vi "DM Message Loop.vi"(8 "error in (no error)":errorcluster, 9 "Data Queue":refnum<queue>, 10 "Data Notifier":refnum<notifier>, 11 "Message Queues":T1) -> (0 "error out":errorcluster)   [LabVIEW 2015, in "DM.lvlib"]
uses:
  DM.lvlib
  support/Message Queue/All Message Queues.ctl
  support/Message Queue/Message Cluster.ctl
  DM Configuration.ctl
  DM State.ctl
  DM Loop State.ctl
  <vilib>/Utility/error.llb/Error Cluster From Error Code.vi
  <vilib>/Utility/file.llb/Read Delimited Spreadsheet (DBL).vi
  <vilib>/ErrorRing/Error Ring.xnode
  support/Message Queue/Message Queue.lvlib
  <userlib>/BMC/BMC.lvlib
panel:
  out "file (use dialog)":path=path "X:/Lab/Equipment/Boston Micromachines Multi-DM/Flash-Drive Contents/C187W147#040_Flat_Map/18W147#040_CLOSED_LOOP_VOLTAGES.txt"
  out "Intensity Graph":dbl[][](graph)
  in  "blank":dbl[](array[slide]) scale=-1.0..1.0
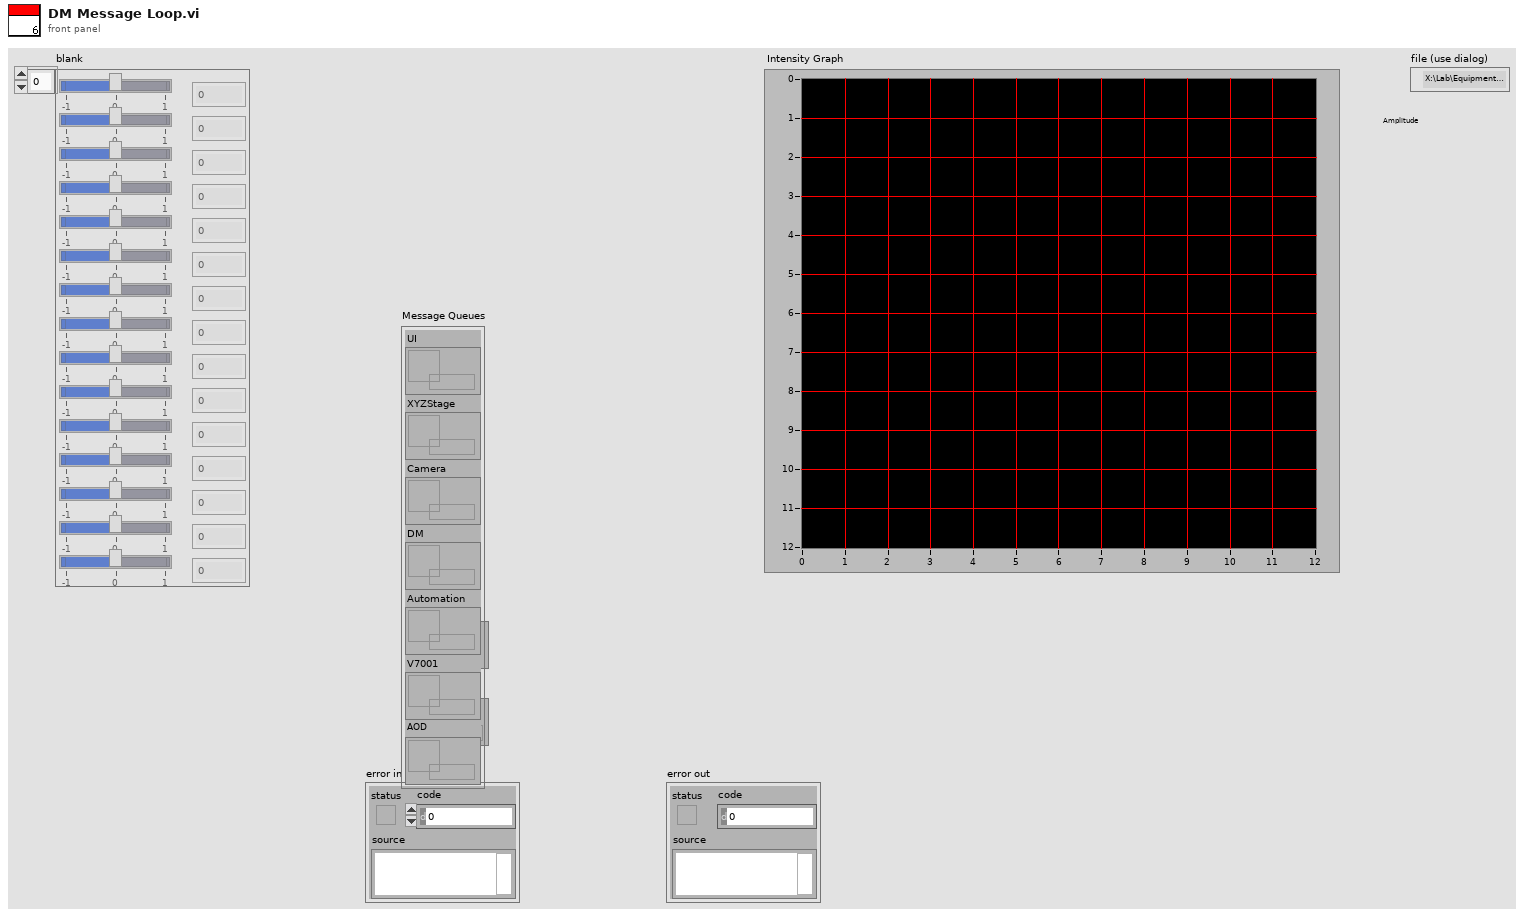
[diagram p1: front panel]
types:
  T1 = typedef "Message Queue.lvlib/All Message Queues.ctl" = cluster{"UI":refnum<queue>, "XYZStage":refnum<queue>, "Camera":refnum<queue>, "DM":refnum<queue>, "Automation":refnum<queue>, "V7001":refnum<queue>, "AOD":refnum<queue>}
  T2 = typedef "DM.lvlib/DM State.ctl" = cluster{"DM State":T3, "Last Image Sent":dbl[][], "Flatmap":dbl[], "Flatmap Path":path, "Matlab Directory Path":path}
  T3 = typedef "DM.lvlib/DM Loop State.ctl" = enum16{"Idle", "Connected"}
  T4 = typedef "DM.lvlib/DM Configuration.ctl" = cluster{"Selected Profile":string, "dm out":cluster{"type":i32, "ID":i32, "size":i32, "@dummy control@":i8, "@dummy control@":i8, "@dummy control@":i8, "@dummy control@":i8, "lutName":u64}}
  T5 = cluster{"type":i32, "ID":i32, "size":i32, "@dummy control@":i8, "@dummy control@":i8, "@dummy control@":i8, "@dummy control@":i8, "lutName":u64}
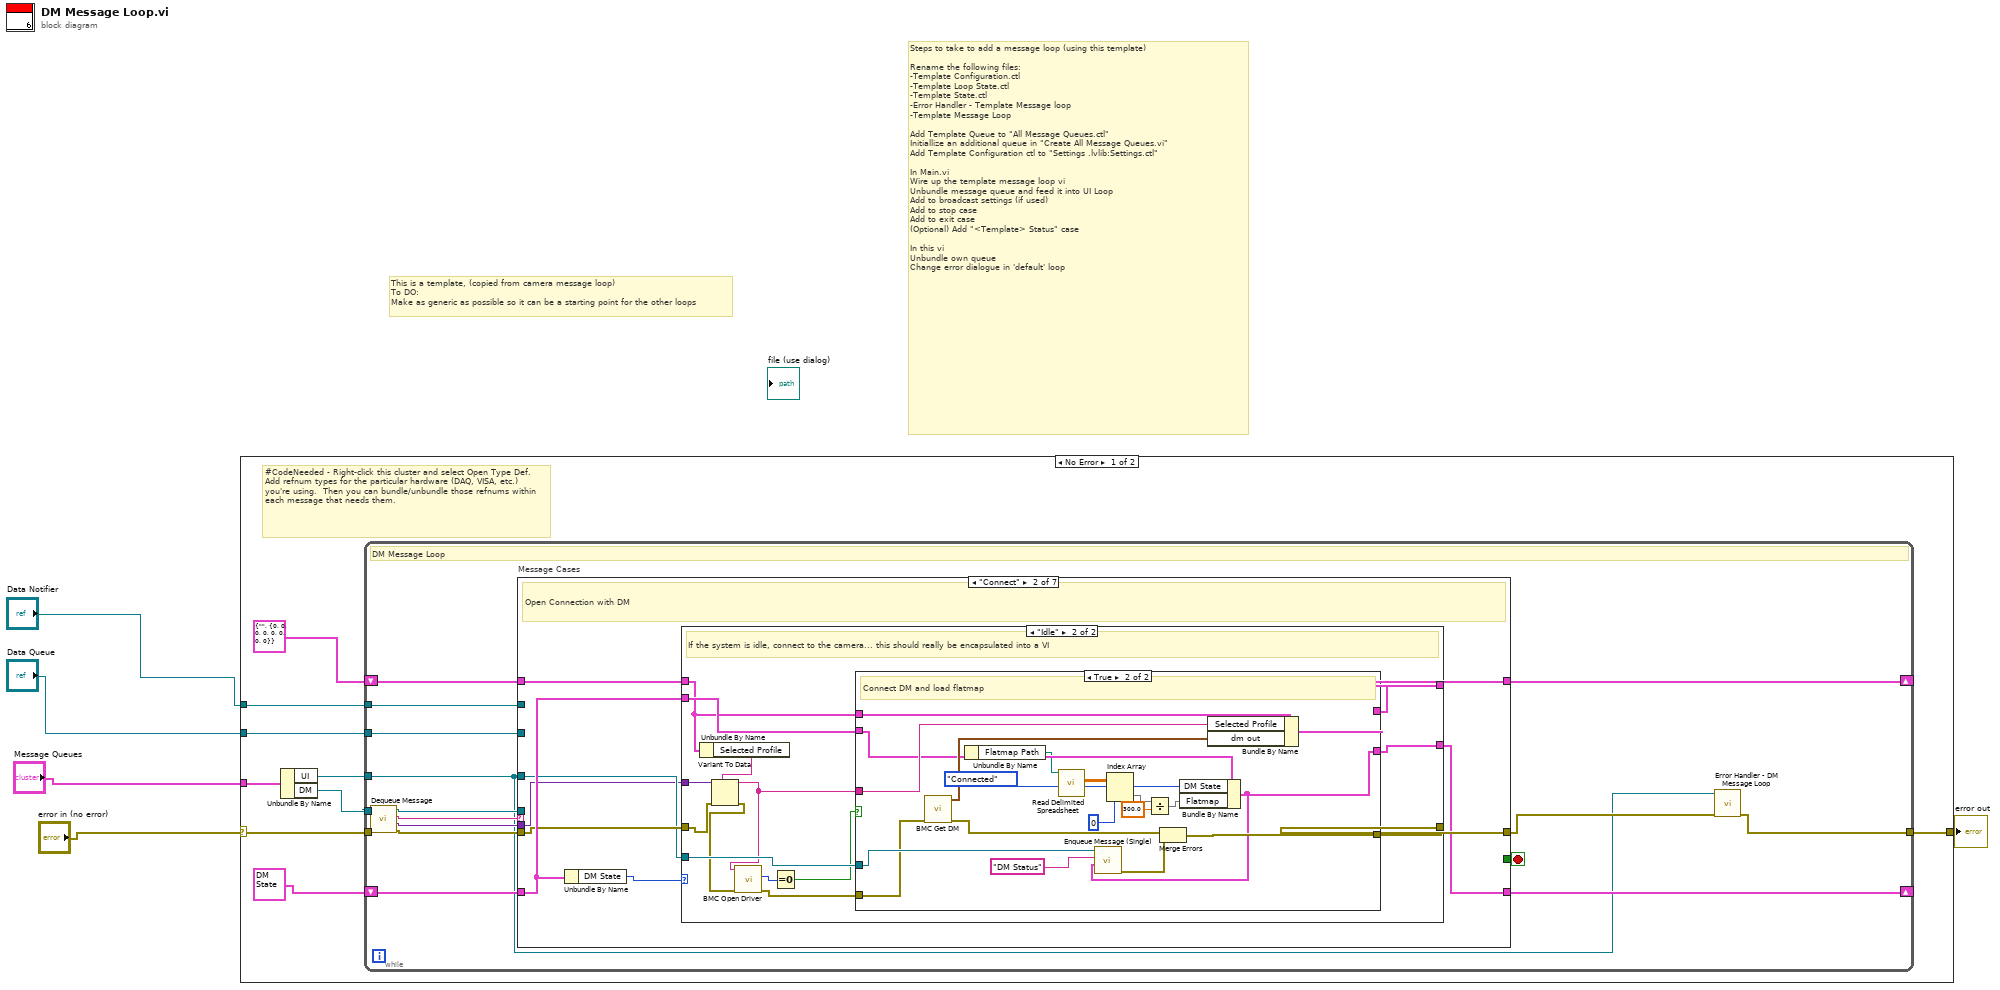
[diagram p0: block diagram]
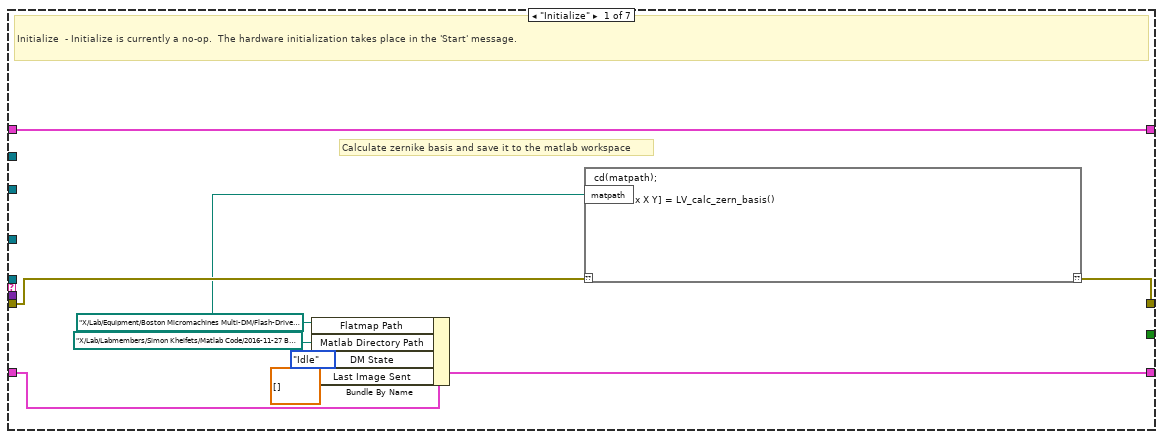
[diagram p2: hidden frame]
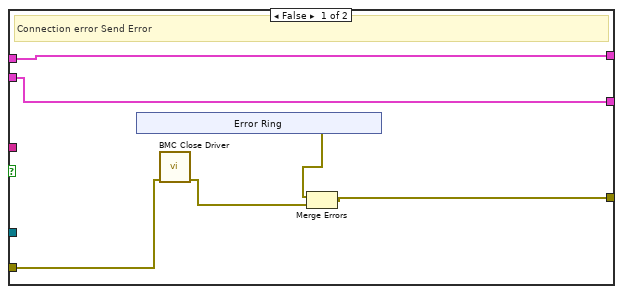
[diagram p4: hidden frame]
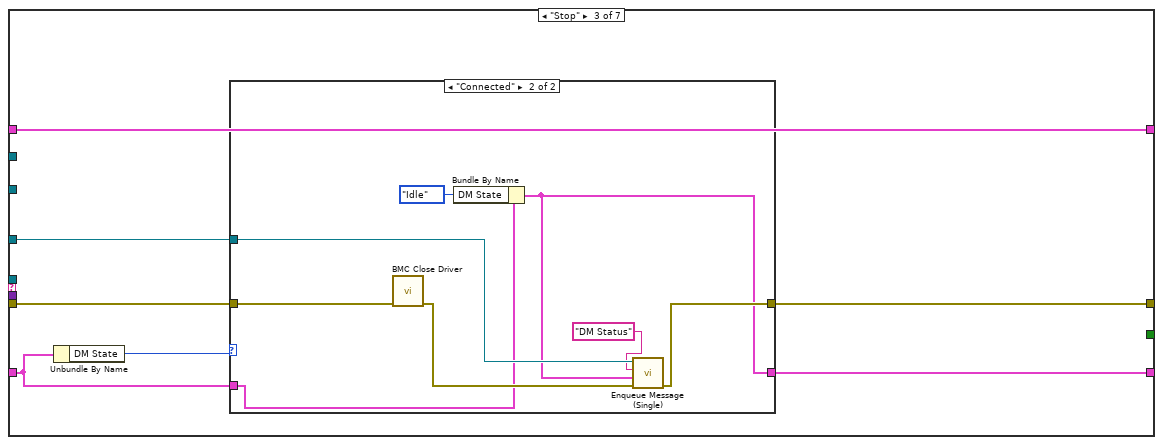
[diagram p5: hidden frame]
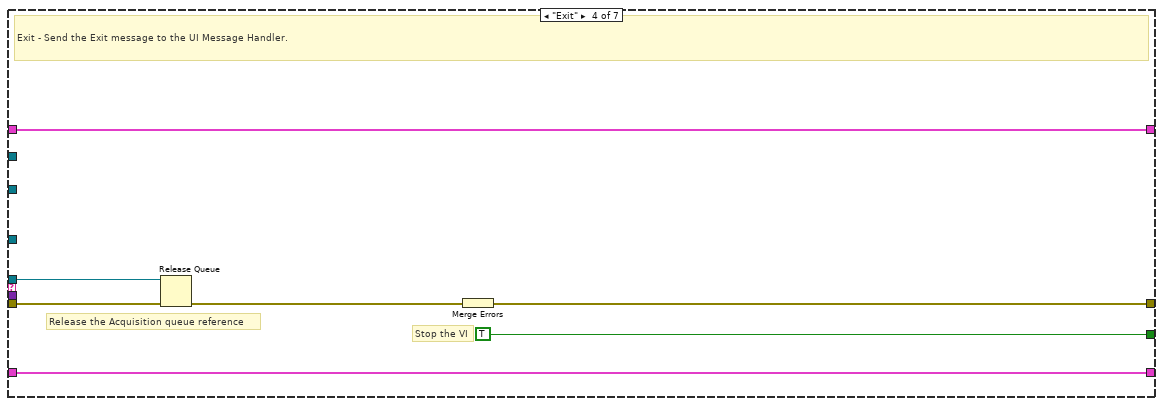
[diagram p7: hidden frame]
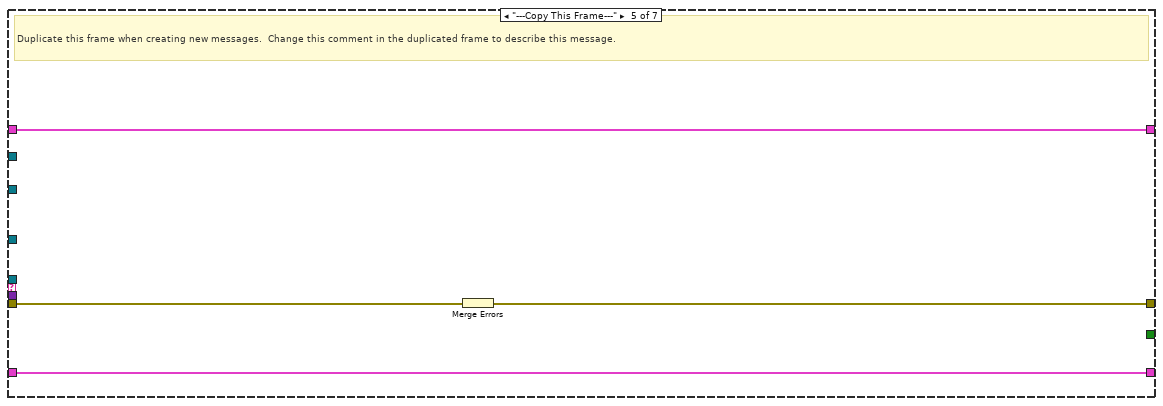
[diagram p8: hidden frame]
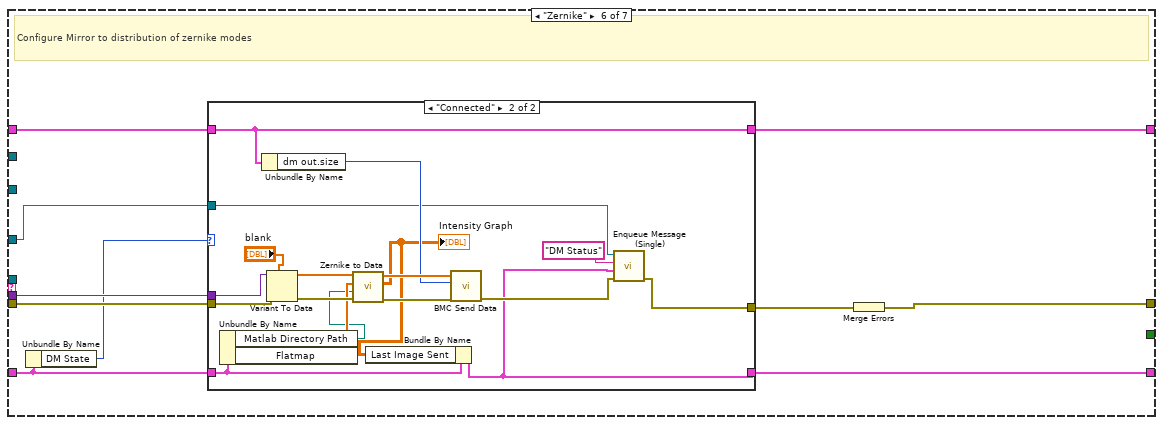
[diagram p9: hidden frame]
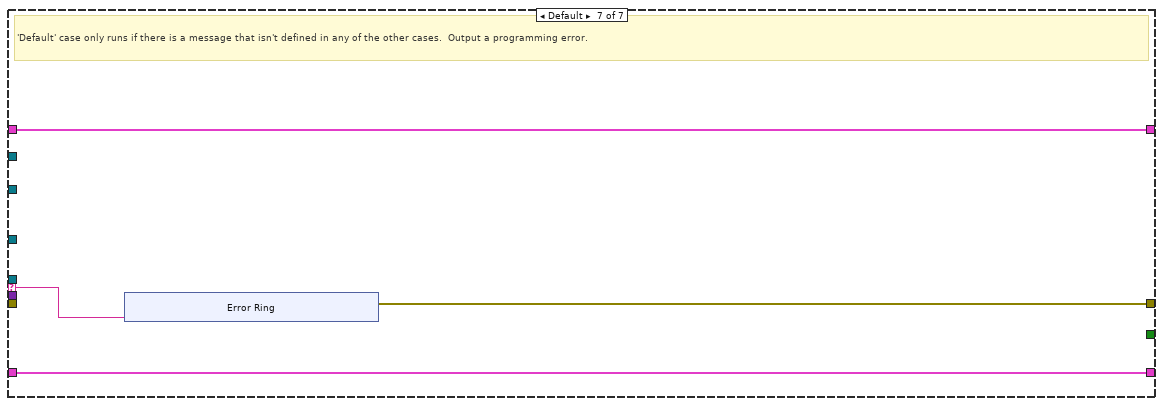
[diagram p11: hidden frame]
diagram:
  # "Steps to take to add a message loop (using this template)\n\nRename the following files:\n-Template Configuration.ctl\n-Template Loop State.ctl\n-Template State.ctl\n-Error Handler - Template Message loop\n-Template Message Loop\n\nAdd Template Queue to \"All Message Queues.ctl\"\nInitiallize an additional queue in \"Create All Message Queues.vi\"\nAdd Template Configuration ctl to \"Settings .lvlib:Settings.ctl\"\n\nIn Main.vi\nWire up the template message loop vi\nUnbundle message queue and feed it into UI Loop\nAdd to broadcast settings (if used)\nAdd to stop case\nAdd to exit case\n(Optional) Add \"<Template> Status\" case\n\nIn this vi\nUnbundle own queue\nChange error dialogue in 'default' loop"
  # "This is a template, (copied from camera message loop)\nTo DO:\nMake as generic as possible so it can be a starting point for the other loops"
  n1 = case shown="No Error" "error in (no error)" {
    selector: "error in (no error)" -> [w11 w166]
    tunnel: "Message Queues" -> [w14 _]
    tunnel: [w12 w166] -> w5
    tunnel: "Data Notifier" -> [w9 _]
    tunnel: "Data Queue" -> [w8 _]
    frame No Error {
      # "#CodeNeeded - Right-click this cluster and select Open Type Def.  Add refnum types for the particular hardware (DAQ, VISA, etc.) you're using.  Then you can bundle/unbundle those refnums within each message that needs them."
      n2 = Unbundle By Name(w14) -> ("UI"=w10:refnum<queue>, "DM"=w13:refnum<queue>)
      n3 = while {
        tunnel: w13 -> [w23]
        shift-right: [w29] -> _
        shift-left: T4 {"Selected Profile"="", "dm out"={"type"=0, "ID"=0, "size"=0, "@dummy control@"=0, "@dummy control@"=0, "@dummy control@"=0, "@dummy control@"=0, "lutName"=0}} ("Hardware Configuration") -> [w30]
        tunnel: w10 -> [w15]
        tunnel: w9 -> [w27]
        tunnel: w8 -> [w26]
        shift-right: [w24] -> _
        shift-left: T2 {"DM State"=enum."Idle", "Last Image Sent"=[], "Flatmap"=[], "Flatmap Path"=path "X:/Lab/Equipment/Boston Micromachines Multi-DM/Flash-Drive Contents/C187W147#040_Flat_Map/18W147#040_CLOSED_LOOP_VOLTAGES.txt", "Matlab Directory Path"=path "X:/Lab/Equipment/Boston Micromachines Multi-DM/Flash-Drive Contents/C187W147#040_Flat_Map/18W147#040_CLOSED_LOOP_VOLTAGES.txt"} ("Cluster") -> [w25]
        tunnel: w11 -> [w22]
        tunnel: [w17] -> w12
        stop <- w28 stop-if-true
        # "DM Message Loop"
        n4 = call "Dequeue Message.vi"("error in (no error)"=w22, "Message Queue"=w23) -> ("error out"=w18:errorcluster, "Message Data"=w19:variant, "Message"=w20:string, "dup Message Queue"=w21:refnum<queue>)  [unwired: 6 in]
        n5 = case "Message Cases" shown="\"Connect\"" w20 {
          selector: w20 -> [_ _ _ _ _ _ w155]
          tunnel: w21 -> [_ _ _ w114 _ _ _]
          tunnel: w18 -> [w34 w45 w100 w116 w123 w131 _]
          tunnel: [w35 w46 w99 w118 w121 w133 w156] -> w16
          tunnel: w30 -> [w39 w44 w102 w117 w122 w130 w158]
          tunnel: [w39 w42 w102 w117 w122 w126 w158] -> w29
          tunnel: [_ _ _ TRUE _ _ _] -> w28
          tunnel: w19 -> [_ w40 _ _ _ w132 _]
          tunnel: w15 -> [_ w41 w98 _ _ w124 _]
          tunnel: w27 -> [_ _ _ _ _ _ _]
          tunnel: w26 -> [_ _ _ _ _ _ _]
          tunnel: w25 -> [w33 w47 w96 w113 w120 w128 w157]
          tunnel: [w38 w43 w97 w113 w120 w129 w157] -> w24
          frame "Initialize" {
            w31 = path "X:/Lab/Labmembers/Simon Kheifets/Matlab Code/2016-11-27 BMC Multi-DM" ("Matlab Directory Path")
            # "Calculate zernike basis and save it to the matlab workspace"
            # "Initialize  - Initialize is currently a no-op.  The hardware initialization takes place in the 'Start' message."
            n6 = Bundle By Name(cluster=w33, "Flatmap Path"=path "X:/Lab/Equipment/Boston Micromachines Multi-DM/Flash-Drive Contents/C187W147#040_Flat_Map/18W147#040_CLOSED_LOOP_VOLTAGES.txt", "Matlab Directory Path"=w31, "DM State"=DM_Loop_State."Idle", "Last Image Sent"=dbl[][] []) -> (w38:T2)
            n7 = script code="cd(matpath);\n\n[basis idx X Y] = LV_calc_zern_basis()"("??"=w34, "matpath"=w31) -> ("??"=w35:errorcluster)
          }
          frame "Connect" {
            # "Open Connection with DM"
            n8 = Unbundle By Name(w47) -> ("DM State"=w48:T3)
            n9 = case shown="\"Idle\"" w48 {
              tunnel: [w51 w65] -> w46
              tunnel: w44 -> [w49 w57]
              tunnel: w45 -> [w51 w54]
              tunnel: [w49 w64] -> w42
              tunnel: [w50 w63] -> w43
              tunnel: w41 -> [_ w62]
              tunnel: w47 -> [w50 w61]
              tunnel: w40 -> [_ w55]
              frame "Connected" {
                # "The system is already acquiring. Ignore the \"Connect\" message."
              }
              frame "Idle" {
                # "If the system is idle, connect to the camera... this should really be encapsulated into a VI"
                n10 = Unbundle By Name(w57) -> ("Selected Profile"=w56:string)
                n11 = Variant To Data(error in=w54, type=w56, Variant=w55) -> (data=w52:string, error out=w53:errorcluster)
                n12 = call <userlib>:"BMC Open Driver.vi"("error in (no error)"=w53, "serial_number"=w52) -> ("error out"=w58:errorcluster, "function return"=w60:i32)  [unwired: 7 in, 1 out]
                n13 = Equal To 0?(x=w60) -> (x = 0?=w59:bool)
                n14 = case shown="True" w59 {
                  tunnel: [w69 w95] -> w65
                  tunnel: w58 -> [w66 w88]
                  tunnel: w57 -> [w71 w87]
                  tunnel: [w71 w86] -> w64
                  tunnel: [w68 w91] -> w63
                  tunnel: w62 -> [_ w94]
                  tunnel: w61 -> [w68 w81]
                  tunnel: w52 -> [_ w84]
                  frame False {
                    # "Connection error Send Error"
                    n15 = xnode "Error Ring"() -> ("error out"=w70:errorcluster)
                    n16 = call <userlib>:"BMC Close Driver.vi"("error in (no error)"=w66) -> ("error out"=w67:errorcluster)  [unwired: 9 in, 1 out]
                    n17 = Merge Errors(w70, w67) -> (w69:errorcluster)
                  }
                  frame True {
                    # "Connect DM and load flatmap"
                    n18 = call <userlib>:"BMC Get DM.vi"("error in (no error)"=w88) -> ("error out"=w89:errorcluster, "dm out"=w85:T5)  [unwired: 7 in, 2 out]
                    n19 = Unbundle By Name(w81) -> ("Flatmap Path"=w80:path)
                    n20 = call-poly <vilib>:"Read Delimited Spreadsheet.vi"("file path (dialog if empty)"=w80) -> ("all rows"=w83:dbl[][])  [unwired: 9 in, 5 out]
                    n21 = Index Array(array=w83, index (col)=0 ("disabled index (col)")) -> (element=w78:dbl[])  [unwired: 1 in]
                    n22 = Divide(x=w78, y=300.0) -> (x/y=w77:dbl[])
                    n23 = Bundle By Name(cluster=w81, "DM State"=DM_Loop_State."Connected", "Flatmap"=w77) -> (w91:T2)
                    n24 = call "Enqueue Message (Single).vi"("Message Data"=w91, "Message"="DM Status", "Message Queue"=w94) -> ("error out"=w92:errorcluster)  [unwired: 7 in, 1 out]
                    n25 = Merge Errors(w89, w92) -> (w95:errorcluster)
                    n26 = Bundle By Name(cluster=w87, "Selected Profile"=w84, "dm out"=w85) -> (w86:T4)
                  }
                }
              }
            }
          }
          frame "Stop" {
            n27 = Unbundle By Name(w96) -> ("DM State"=w101:T3)
            n28 = case shown="\"Connected\"" w101 {
              tunnel: w100 -> [w104 w112]
              tunnel: [w104 w110] -> w99
              tunnel: w98 -> [_ w109]
              tunnel: [w103 w105] -> w97
              tunnel: w96 -> [w103 w107]
              frame "Idle", Default {
                # "If disconnected, do nothing"
              }
              frame "Connected" {
                n29 = call <userlib>:"BMC Close Driver.vi"("error in (no error)"=w112) -> ("error out"=w111:errorcluster)  [unwired: 9 in, 1 out]
                n30 = Bundle By Name(cluster=w107, "DM State"=DM_Loop_State."Idle") -> (w105:T2)
                n31 = call "Enqueue Message (Single).vi"("error in (no error)"=w111, "Message Data"=w105, "Message"="DM Status", "Message Queue"=w109) -> ("error out"=w110:errorcluster)  [unwired: 6 in, 1 out]
              }
            }
          }
          frame "Exit" {
            # "Release the Acquisition queue reference"
            # "Stop the VI"
            # "Exit - Send the Exit message to the UI Message Handler."
            n32 = Release Queue(queue=w114, error in (no error)=w116) -> (error out=w115:errorcluster)  [unwired: 1 in, 2 out]
            n33 = Merge Errors(w115) -> (w118:errorcluster)
          }
          frame "---Copy This Frame---" {
            # "Duplicate this frame when creating new messages.  Change this comment in the duplicated frame to describe this message."
            n34 = Merge Errors(w123) -> (w121:errorcluster)
          }
          frame "Zernike" {
            # "Configure Mirror to distribution of zernike modes"
            n35 = Unbundle By Name(w128) -> ("DM State"=w127:T3)
            n36 = case shown="\"Connected\"" w127 {
              tunnel: w132 -> [_ w154]
              tunnel: w131 -> [w134 w153]
              tunnel: w130 -> [w136 w140]
              tunnel: [w135 w142] -> w129
              tunnel: w128 -> [w135 w139]
              tunnel: [w136 w140] -> w126
              tunnel: [w134 w145] -> w125
              tunnel: w124 -> [_ w141]
              frame "Idle", Default {
              }
              frame "Connected" {
                n37 = Unbundle By Name(w139) -> ("Matlab Directory Path"=w137:path, "Flatmap"=w138:dbl[])
                n38 = Unbundle By Name(w140) -> ("dm out.size"=w147:i32)
                n39 = Variant To Data(error in=w153, type="blank", Variant=w154) -> (data=w151:dbl[], error out=w150:errorcluster)
                n40 = call "Zernike to Data.vi"("error in (no error)"=w150, "Matlab Directory Path"=w137, "Flatmap"=w138, "Zernike modes in"=w151) -> ("error out"=w148:errorcluster, "2D Data Out"=w146:dbl[][], "1D Data Out"=w149:dbl[])  [unwired: 5 in]
                "Intensity Graph" <- w146
                n41 = Bundle By Name(cluster=w139, "Last Image Sent"=w146) -> (w142:T2)
                n42 = call <userlib>:"BMC Send Data.vi"("error in (no error)"=w148, "length"=w147, "data"=w149) -> ("error out"=w144:errorcluster)  [unwired: 6 in, 2 out]
                n43 = call "Enqueue Message (Single).vi"("error in (no error)"=w144, "Message Data"=w142, "Message"="DM Status", "Message Queue"=w141) -> ("error out"=w145:errorcluster)  [unwired: 6 in, 1 out]
              }
            }
            n44 = Merge Errors(w125) -> (w133:errorcluster)
          }
          frame Default {
            # "'Default' case only runs if there is a message that isn't defined in any of the other cases.  Output a programming error."
            n45 = xnode "Error Ring"("parameter 0"=w155) -> ("error out"=w156:errorcluster)
          }
        }
        n46 = call "Error Handler - DM Message Loop.vi"("error in (no error)"=w16, "Message Queue"=w15) -> ("dup error in"=w17:errorcluster)  [unwired: 8 in, 1 out]
      }
    }
    frame Error {
    }
  }
  "error out" <- w5
